vi "Turn Calc.vi"(0 "Desired Angle (radians)":dbl, 1 "Reverse":bool, 2 "Tolerance":dbl=0.08, 3 "Base":dbl=0.6, 4 "Ratio":dbl=0.25 format="%#_13g", 6 "Drive Tol":dbl=0.5) -> (14 "Drive X Output":dbl, 15 "Adjusted Angle":dbl, 18 "Drive In Range?":bool, 19 "In Range?":bool)   [LabVIEW 2016]
doc: "outside of range: base (lowest speed) + ratio (how much higher than base it is) * distance (radians)\n(determines how fast to turn if out of range)\n\nin range: output 0 (do nothing)\n\ndrive x output: wire into arcade drive block for x\n\ndrive tolerance: how much it can be off before driving forward"
uses:
  Robot Global Data.vi
panel:
  in  "Max Min":dbl=1.0
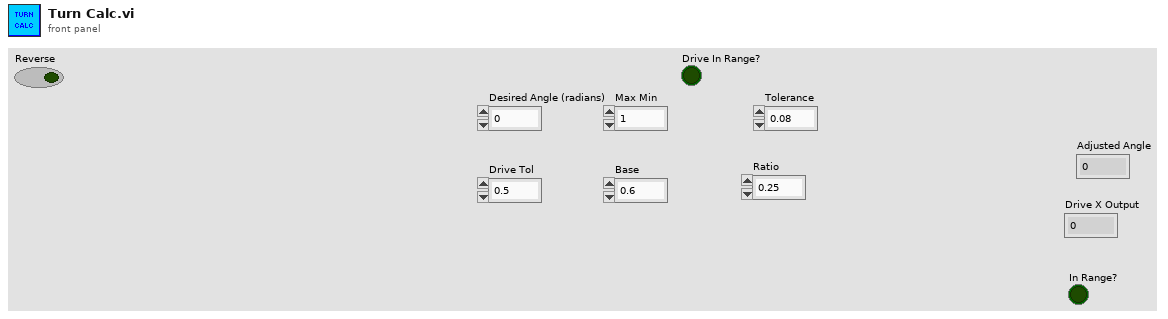
[diagram p1: front panel]
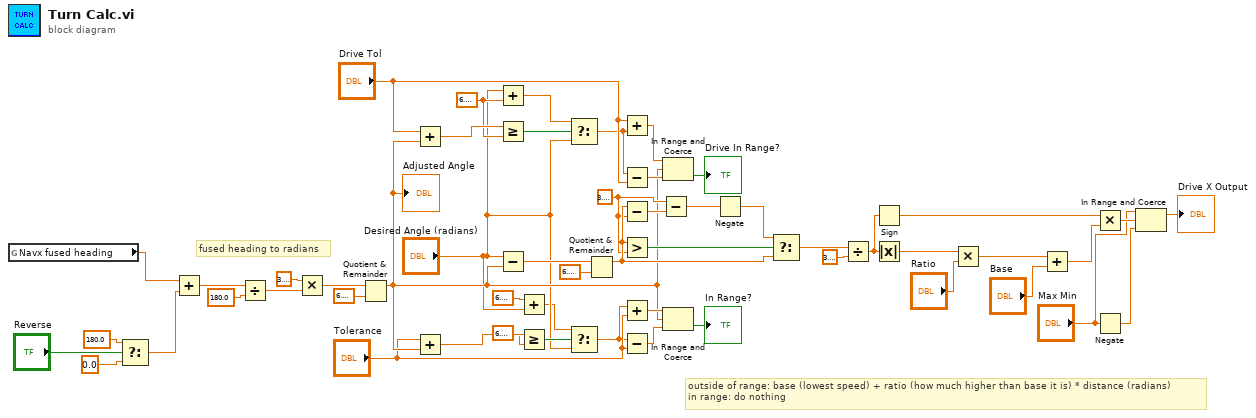
[diagram p0: block diagram]
diagram:
  w12 = 6.283185307179586
  w20 = 3.141592653589793
  # "fused heading to radians"
  # "outside of range: base (lowest speed) + ratio (how much higher than base it is) * distance (radians)\nin range: do nothing"
  n1 = global read "Robot Global Data.vi" "Navx fused heading"() -> (w1:dbl)
  n2 = Select(t=180.0 ("y"), s="Reverse", f=0.0) -> (s? t:f=w23:dbl)
  n3 = Add(x=w1, y=w23) -> (x+y=w28:dbl)
  n4 = Divide(x=w28, y=180.0) -> (x/y=w34:dbl)
  n5 = Multiply(x=3.141592653589793, y=w34) -> (x*y=w33:dbl)
  n6 = Quotient & Remainder(x=w33, y=6.283185307179586) -> (x-y*floor(x/y)=w7:dbl)  [unwired: 1 out]
  "Adjusted Angle" <- w7
  n7 = Add(x="Drive Tol", y=w7) -> (x+y=w15:dbl)
  n8 = Add(x="Tolerance", y=w7) -> (x+y=w10:dbl)
  n9 = Add(x="Desired Angle (radians)", y=w12) -> (x+y=w13:dbl)
  n10 = Greater Or Equal?(x=w15, y=w12) -> (x >= y?=w14:bool)
  n11 = Subtract(x="Desired Angle (radians)", y=w7) -> (x-y=w51:dbl)
  n12 = Add(x=6.283185307179586, y="Desired Angle (radians)") -> (x+y=w3:dbl)
  n13 = Greater Or Equal?(x=w10, y=6.283185307179586) -> (x >= y?=w9:bool)
  n14 = Select(t=w13, s=w14, f="Desired Angle (radians)") -> (s? t:f=w11:dbl)
  n15 = Select(t=w3, s=w9, f="Desired Angle (radians)") -> (s? t:f=w2:dbl)
  n16 = Quotient & Remainder(x=w51, y=6.283185307179586) -> (x-y*floor(x/y)=w49:dbl)  [unwired: 1 out]
  n17 = Add(x="Drive Tol", y=w11) -> (x+y=w17:dbl)
  n18 = Subtract(x=w11, y="Drive Tol") -> (x-y=w18:dbl)
  n19 = Subtract(x=w49, y=w20) -> (x-y=w29:dbl)
  n20 = Greater?(x=w49, y=w20) -> (0:w31:bool)
  n21 = Add(x=w2, y="Tolerance") -> (x+y=w48:dbl)
  n22 = Subtract(x=w2, y="Tolerance") -> (x-y=w47:dbl)
  n23 = Subtract(x=w20, y=w29) -> (x-y=w30:dbl)
  n24 = In Range and Coerce(upper limit=w17, x=w7, lower limit=w18) -> (In Range?=→"Drive In Range?":bool)  [unwired: 1 out]
  n25 = In Range and Coerce(upper limit=w48, x=w7, lower limit=w47) -> (In Range?=→"In Range?":bool)  [unwired: 1 out]
  n26 = Negate(x=w30) -> (-x=w32:dbl)
  n27 = Select(t=w32, s=w31, f=w49) -> (s? t:f=w37:dbl)
  n28 = Divide(x=w37, y=3.141592653589793) -> (x/y=w36:dbl)
  n29 = Sign(1:w36) -> (0:w42:dbl)
  n30 = Absolute Value(x=w36) -> (abs(x)=w43:dbl)
  n31 = Multiply(x=w43, y="Ratio") -> (x*y=w45:dbl)
  n32 = Add(x=w45, y="Base") -> (x+y=w38:dbl)
  n33 = Multiply(x=w42, y=w38) -> (x*y=w41:dbl)
  n34 = Negate(x="Max Min") -> (-x=w40:dbl)
  n35 = In Range and Coerce(upper limit="Max Min", x=w41, lower limit=w40) -> (coerced(x)=→"Drive X Output":dbl)  [unwired: 1 out]
